vi "Write Tx Root Content Msg.vi"(10 "Nested Actor.lvlib:Tx Root Content Msg.lvclass":refnum<class "Tx Root Content Msg.lvclass">, 11 "Nested Actor in":refnum<class "Nested Actor.lvclass">) -> (3 "Nested Actor out":refnum<class "Nested Actor.lvclass">)   [LabVIEW 2020, in "Nested Actor.lvlib" / "Nested Actor.lvclass"]
uses:
  Nested Actor.lvclass
  Nested Actor Messages/Tx Root Content Msg/Tx Root Content Msg.lvclass
  Nested Actor.lvclass/Nested Actor.ctl
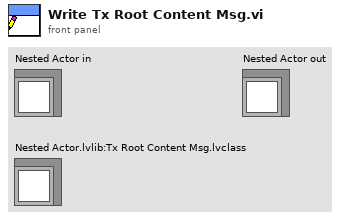
[diagram p1: front panel]
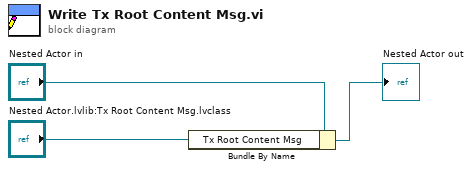
[diagram p0: block diagram]
diagram:
  n1 = Bundle By Name(cluster="Nested Actor in", "Tx Root Content Msg"="Nested Actor.lvlib:Tx Root Content Msg.lvclass") -> (→"Nested Actor out":refnum<class "Nested Actor.lvclass">)
